vi "TreeNode Make Timestamped Segment.vi"(0 "TreeNode DVR in":refnum<data-value>, 5 "Segment Data DVR":refnum<data-value>, 7 "Timestamps":i64[](array[numeric]), 11 "error in (no error)":errorcluster) -> (4 "TreeNode DVR out":refnum<data-value>, 15 "error out":errorcluster)   [LabVIEW 2015, in "MDSplus.lvlib"]
doc: "Write a single row of timestamped data."
uses:
  <vilib>/MDSplus/Library/MDSplus.lvlib
  <vilib>/MDSplus/Classes/Data_Class/TreeNode_Class/TreeNode.lvclass
  <vilib>/MDSplus/Classes/Data_Class/Data.lvclass
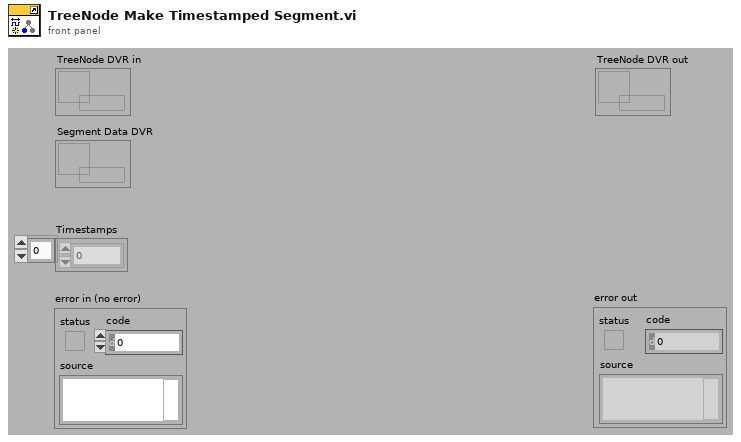
[diagram p1: front panel]
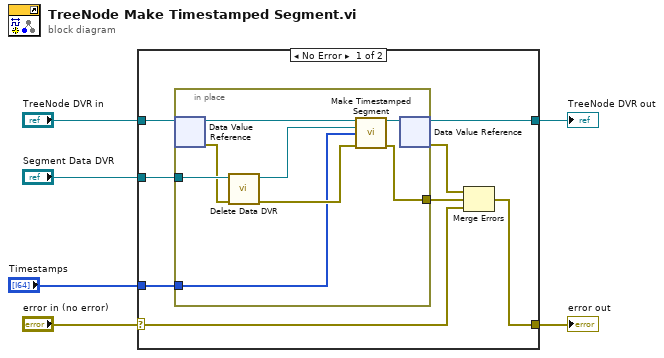
[diagram p0: block diagram]
diagram:
  n1 = case shown="No Error" "error in (no error)" {
    selector: "error in (no error)" -> [w13 w23]
    tunnel: "TreeNode DVR in" -> [w14 w24]
    tunnel: [w10 w23] -> w6
    tunnel: [w11 w24] -> w3
    tunnel: "Segment Data DVR" -> [w8 _]
    tunnel: "Timestamps" -> [w7 _]
    frame No Error {
      n2 = in-place {
        in-place-border: [w18] -> w9
        in-place-border: w8 -> [w22]
        in-place-border: w7 -> [w15]
        n3 = in-place-dvr #1(w14) -> (w20:refnum<class "TreeNode.lvclass">, w21:errorcluster)
        n4 = call <vilib>:"Delete Data DVR.vi"("error in (no error)"=w21, "Data DVR in"=w22) -> ("error out"=w16:errorcluster, "Data out"=w17:refnum<class "Data.lvclass">)  [unwired: 8 in]
        n5 = call-dynamic "Make Timestamped Segment.vi"("TreeNode in"=w20, "Segment data"=w17, "Timestamps"=w15, "error in (no error)"=w16) -> ("TreeNode out"=w19:refnum<class "TreeNode.lvclass">, "error out"=w18:errorcluster)  [unwired: 10 in]
        n6 = in-place-dvr #1(w19) -> (w11:refnum<data-value>, w12:errorcluster)
      }
      n7 = Merge Errors(w12, w9, w13) -> (w10:errorcluster)
    }
    frame Error {
    }
  }
  "error out" <- w6
  "TreeNode DVR out" <- w3
